vi "CRYOptional Modules.vi"() -> ()   [LabVIEW 2013]
doc: "Config File Reading/Writting\n\nPath \n ini File path\nRWFlag\n 0: no action\n 1: read\n 2: write"
panel:
  in  "Draw":bool
  in  "Modules List":i32[](listbox)
  in  "OK":bool
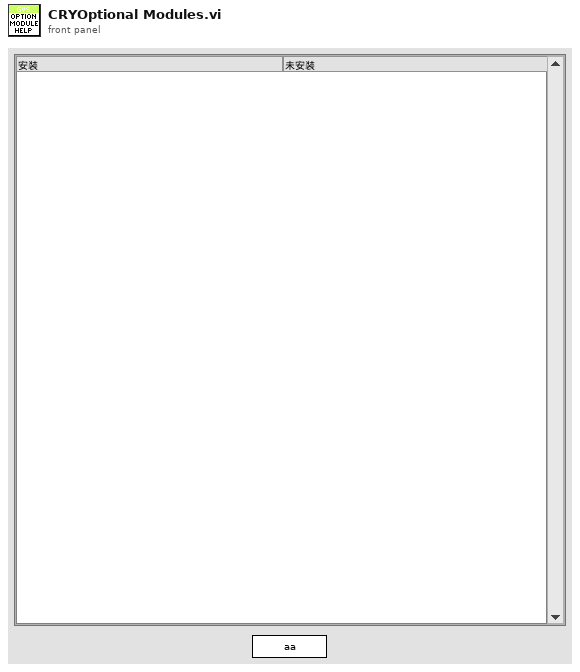
[diagram p1: front panel]
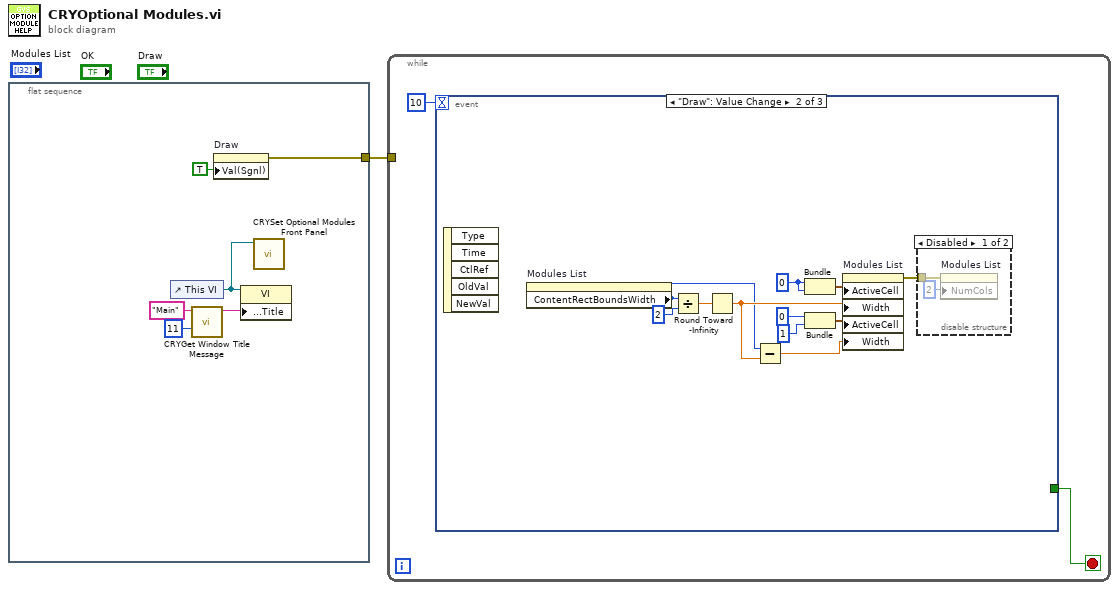
[diagram p0: block diagram]
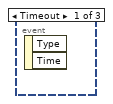
[diagram p2: hidden frame]
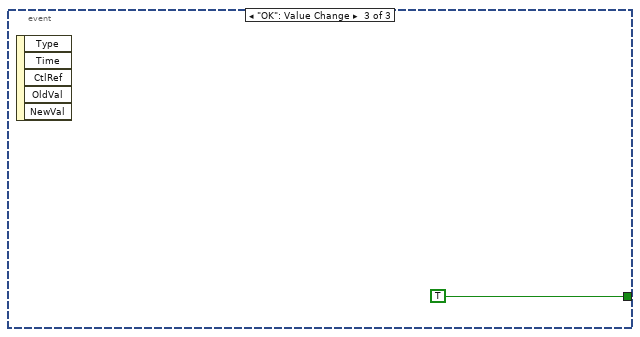
[diagram p4: hidden frame]
diagram:
  n1 = flat-sequence {
    tunnel: [w2] -> w1
    frame #0 {
      n2 = control-ref of="This VI"() -> (w3:refnum<vi>)
      n3 = call "CRYGet Window Title Message.vi"("No"=11 ("Error No"), "Kind"="Main") -> ("Multibyte String"=w4:string)  [unwired: 4 in, 5 out]
      n4 = property on="Draw" class="Bool (strict)"("Val(Sgnl)"=TRUE ("Value (Signaling)")) -> (error out=w2:errorcluster)  [unwired: 2 in, 1 out]
      n5 = property class="VI"(reference=w3, "Front Panel.Title"=w4) -> ()  [unwired: 1 in, 2 out]
      n6 = call "CRYSet Optional Modules Front Panel.vi"("Vi Ref In"=w3) -> ()  [unwired: 10 in, 1 out]
    }
  }
  n7 = while {
    tunnel: w1 -> [_]
    stop <- w8 stop-if-true
    n8 = event shown="[1] \"Draw\": Value Change" {
      selector: _ -> [_ _ _]
      dyn-events: _ -> [_ _ _]
      timeout: 10 -> [_ _ _]
      tunnel: [_ _ TRUE ("NewVal")] -> w8
      event Timeout {
        n9 = event-data() -> ()  [unwired: 1 in, 2 out]
      }
      event "Draw": Value Change {
        w13 = 0 ("Column")
        n10 = event-data() -> ()  [unwired: 1 in, 5 out]
        n11 = property on="Modules List" class="MCListbox (strict)"() -> ("ContentRectBoundsWidth"=w18:i32)  [unwired: 2 in, 2 out]
        n12 = Divide(x=w18, y=u32 2) -> (x/y=w14:dbl)
        n13 = Round Toward -Infinity(1:w14) -> (0:w19:dbl)
        n14 = Subtract(x=w18, y=w19) -> (x-y=w20:dbl)
        n15 = Bundle("Column"=w13, "Column"=w13) -> (w12:cluster{"Column":i32, "Column":i32})  [unwired: 1 in]
        n16 = Bundle("Column"=0, "Column"=1) -> (w16:cluster{"Column":i32, "Column":i32})  [unwired: 1 in]
        n17 = property on="Modules List" class="MCListbox (strict)"("ActiveCell"=w12, "Width"=w19, "ActiveCell"=w16, "Width"=w20) -> (error out=w11:errorcluster)  [unwired: 2 in, 1 out]
        n18 = disable-structure shown="Disabled" {
          disable-tunnel: w11 -> [w21 _]
          frame Disabled {
            n19 = property on="Modules List" class="MCListbox (strict)"(error in=w21, "NumCols"=u32 2 ("Number of Columns")) -> ()  [unwired: 1 in, 2 out]
          }
          frame Enabled {
          }
        }
      }
      event "OK": Value Change {
        n20 = event-data() -> ()  [unwired: 1 in, 5 out]
      }
    }
  }
